vi "mfd_gps.vi"(8 "Refresh Rate (Hz)":u32=5) -> ()   [LabVIEW 2023]
uses:
  mfd_global.vi
panel:
  out "x .or. y?":bool
  out "GPS_RAW_INT":T1
  out "MFD_Gps":picture
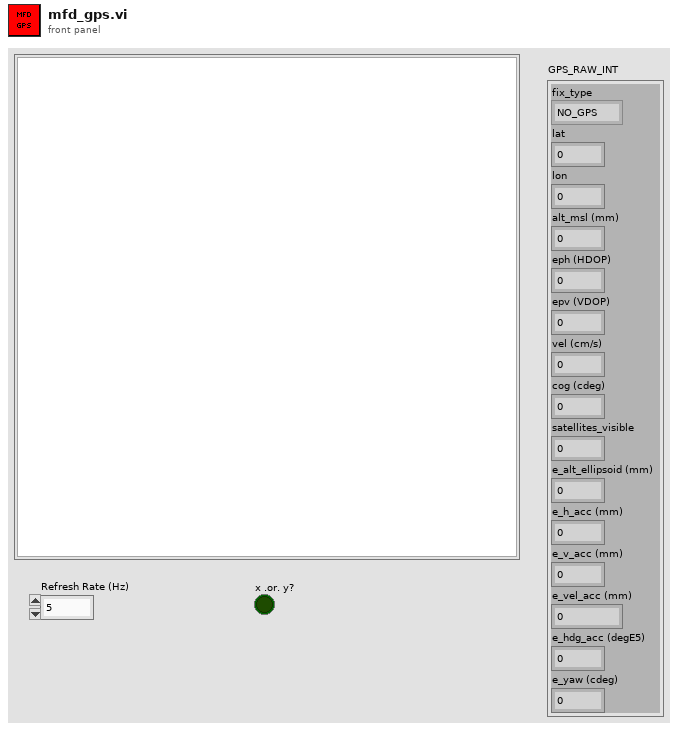
[diagram p1: front panel]
types:
  T1 = cluster{"lat":i32, "lon":i32, "alt_msl (mm)":i32, "eph (HDOP)":u16, "epv (VDOP)":u16, "vel (cm/s)":u16, "cog (cdeg)":u16, "satellites_visible":u8, "e_alt_ellipsoid (mm)":i32, "e_h_acc (mm)":u32, "e_v_acc (mm)":u32, "e_vel_acc (mm)":u32, "e_hdg_acc (degE5)":u32, "e_yaw (cdeg)":u16, "fix_type":enum16{"NO_GPS", "NO_FIX", "2D_FIX", "3D_FIX", "DGPS", "RTK_FLOAT", "RTK_FIXED", "STATIC", "PPP"}}
  T2 = cluster{"left":i16, "top":i16, "right":i16, "bottom":i16}
  T3 = cluster{"Font Name:":string, "Size":i16, "Strikeout?":bool, "Italic?":bool, "Underline?":bool, "Outline?":bool, "Shadow?":bool, "Bold?":bool}
  T4 = enum16{"User-specified Font", "Application Font", "System Font", "Dialog Font"}
  T5 = cluster{"horizontal":enum16{"left", "center", "right"}, "vertical":enum16{"top", "center", "bottom"}}
  T6 = cluster{"Width":u16, "Style":enum32{"Solid", "Dash", "Dot", "DashDot", "DashDotDot"}}
  T7 = typedef "imagedata.ctl" = cluster{"image type":i32, "image depth":i32, "image":u8[], "mask":u8[], "colors":u32[], "Rectangle":cluster{"left":i16, "top":i16, "right":i16, "bottom":i16}}
  T8 = cluster{"lat":bool, "lon":bool, "alt_msl (mm)":bool, "eph (HDOP)":bool, "epv (VDOP)":bool, "vel (cm/s)":bool, "cog (cdeg)":bool, "satellites_visible":bool, "e_alt_ellipsoid (mm)":bool, "e_h_acc (mm)":bool, "e_v_acc (mm)":bool, "e_vel_acc (mm)":bool, "e_hdg_acc (degE5)":bool, "e_yaw (cdeg)":bool, "fix_type":bool}
  T9 = enum16{"NO_GPS", "NO_FIX", "2D_FIX", "3D_FIX", "DGPS", "RTK_FLOAT", "RTK_FIXED", "STATIC", "PPP"}
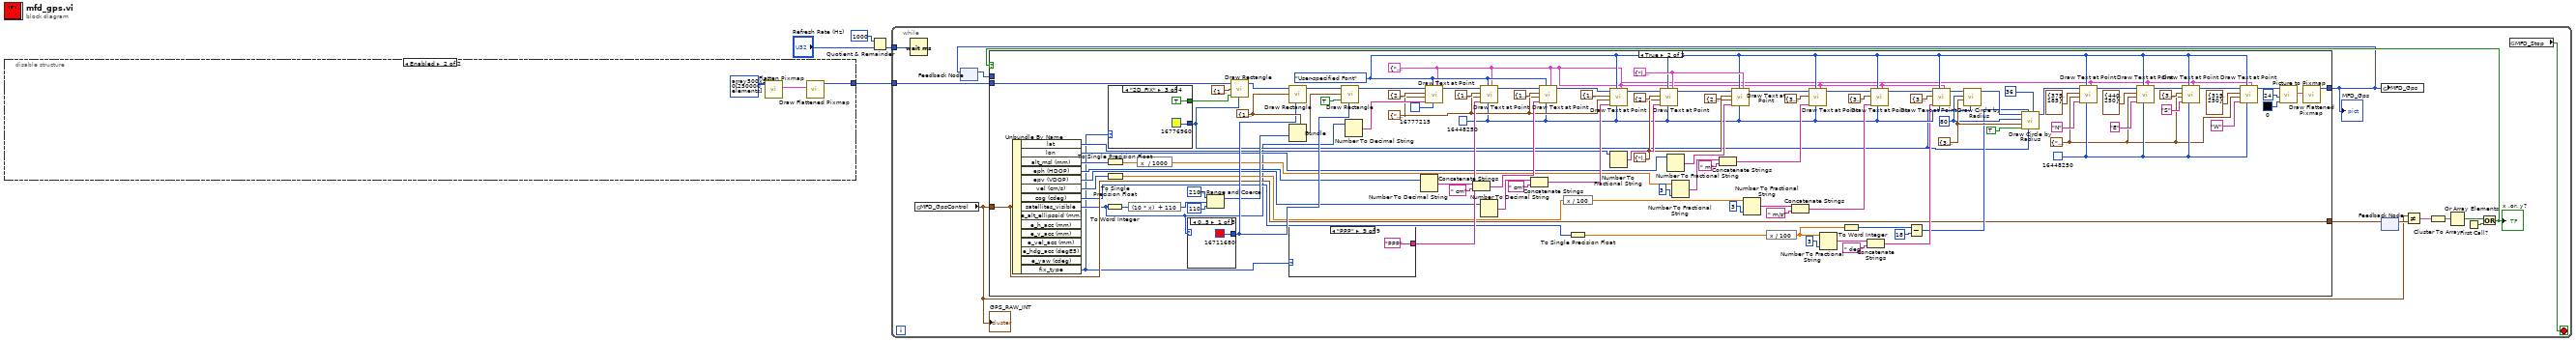
[diagram p0: block diagram]
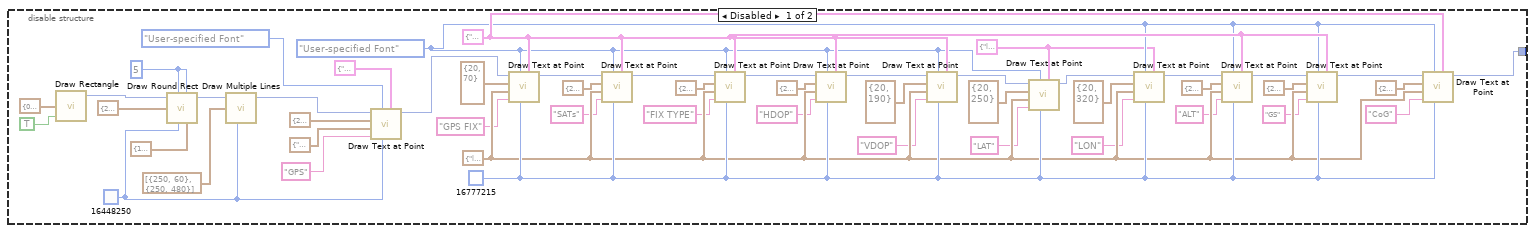
[diagram p2: hidden frame]
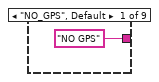
[diagram p4: hidden frame]
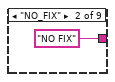
[diagram p5: hidden frame]
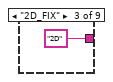
[diagram p6: hidden frame]
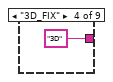
[diagram p7: hidden frame]
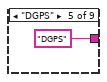
[diagram p8: hidden frame]
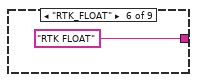
[diagram p9: hidden frame]
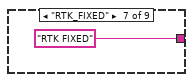
[diagram p10: hidden frame]
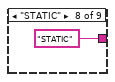
[diagram p11: hidden frame]
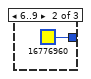
[diagram p12: hidden frame]
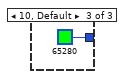
[diagram p13: hidden frame]
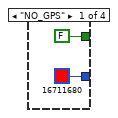
[diagram p14: hidden frame]
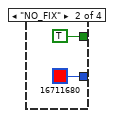
[diagram p15: hidden frame]
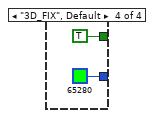
[diagram p16: hidden frame]
diagram:
  n1 = disable-structure shown="Enabled" {
    disable-tunnel: [w5 w56] -> w4
    frame Disabled {
      w32 = T3 {"Font Name:"="latlon", "Size"=21, "Strikeout?"=FALSE, "Italic?"=FALSE, "Underline?"=FALSE, "Outline?"=FALSE, "Shadow?"=FALSE, "Bold?"=TRUE} ("[user-specified font]")
      w38 = T5 {"horizontal"=enum."left", "vertical"=enum."top"} ("alignment(left, top)")
      w42 = T3 {"Font Name:"="gps", "Size"=18, "Strikeout?"=FALSE, "Italic?"=FALSE, "Underline?"=FALSE, "Outline?"=FALSE, "Shadow?"=FALSE, "Bold?"=TRUE} ("[user-specified font]")
      w41 = u32 16777215 ("text color(black)")
      w40 = T4."User-specified Font" ("desired font(Application)")
      w16 = u32 16448250 ("text color(black)")
      w10 = i16 5 ("oval height")
      n2 = call <vilib>:"Draw Rectangle.vi"("rect"=T2 {"left"=0, "top"=0, "right"=500, "bottom"=500}, "fill?(F)"=TRUE) -> ("new picture"=w43:picture)  [unwired: 7 in]
      n3 = call <vilib>:"Draw Round Rect.vi"("picture"=w43, "oval width"=w10, "rect"=T2 {"left"=220, "top"=17, "right"=280, "bottom"=47} ("rect 2"), "color(black)"=w16, "oval height"=w10, "pen"=T6 {"Width"=1, "Style"=enum."Solid"}) -> ("new picture"=w44:picture)  [unwired: 3 in]
      n4 = call <vilib>:"Draw Multiple Lines.vi"("picture"=w44, "line endpoints"=cluster{"x":i16, "y":i16}[] [{"x"=250, "y"=60}, {"x"=250, "y"=480}], "color(black)"=w16) -> ("new picture"=w45:picture)  [unwired: 6 in]
      n5 = call <vilib>:"Draw Text at Point.vi"("[user-specified font]"=T3 {"Font Name:"="r", "Size"=25, "Strikeout?"=FALSE, "Italic?"=FALSE, "Underline?"=FALSE, "Outline?"=FALSE, "Shadow?"=FALSE, "Bold?"=TRUE}, "text color(black)"=w16, "desired font(Application)"=T4."User-specified Font", "text"="GPS", "alignment(left, top)"=T5 {"horizontal"=enum."center", "vertical"=enum."top"}, "origin"=cluster{"x":i16, "y":i16} {"x"=250, "y"=20}, "picture"=w45) -> ("new picture"=w46:picture)  [unwired: 3 in, 1 out]
      n6 = call <vilib>:"Draw Text at Point.vi"("[user-specified font]"=w42, "text color(black)"=w41, "desired font(Application)"=w40, "text"="GPS FIX", "alignment(left, top)"=w38, "origin"=cluster{"x":i16, "y":i16} {"x"=20, "y"=70}, "picture"=w46) -> ("new picture"=w47:picture)  [unwired: 3 in, 1 out]
      n7 = call <vilib>:"Draw Text at Point.vi"("[user-specified font]"=w42, "text color(black)"=w41, "desired font(Application)"=w40, "text"="SATs", "alignment(left, top)"=w38, "origin"=cluster{"x":i16, "y":i16} {"x"=20, "y"=100}, "picture"=w47) -> ("new picture"=w48:picture)  [unwired: 3 in, 1 out]
      n8 = call <vilib>:"Draw Text at Point.vi"("[user-specified font]"=w42, "text color(black)"=w41, "desired font(Application)"=w40, "text"="FIX TYPE", "alignment(left, top)"=w38, "origin"=cluster{"x":i16, "y":i16} {"x"=20, "y"=130} ("origin 2"), "picture"=w48) -> ("new picture"=w49:picture)  [unwired: 3 in, 1 out]
      n9 = call <vilib>:"Draw Text at Point.vi"("[user-specified font]"=w42, "text color(black)"=w41, "desired font(Application)"=w40, "text"="HDOP", "alignment(left, top)"=w38, "origin"=cluster{"x":i16, "y":i16} {"x"=20, "y"=160}, "picture"=w49) -> ("new picture"=w50:picture)  [unwired: 3 in, 1 out]
      n10 = call <vilib>:"Draw Text at Point.vi"("[user-specified font]"=w42, "text color(black)"=w41, "desired font(Application)"=w40, "text"="VDOP", "alignment(left, top)"=w38, "origin"=cluster{"x":i16, "y":i16} {"x"=20, "y"=190}, "picture"=w50) -> ("new picture"=w51:picture)  [unwired: 3 in, 1 out]
      n11 = call <vilib>:"Draw Text at Point.vi"("[user-specified font]"=w32, "text color(black)"=w41, "desired font(Application)"=w40, "text"="LAT", "alignment(left, top)"=w38, "origin"=cluster{"x":i16, "y":i16} {"x"=20, "y"=250}, "picture"=w51) -> ("new picture"=w52:picture)  [unwired: 3 in, 1 out]
      n12 = call <vilib>:"Draw Text at Point.vi"("[user-specified font]"=w32, "text color(black)"=w41, "desired font(Application)"=w40, "text"="LON", "alignment(left, top)"=w38, "origin"=cluster{"x":i16, "y":i16} {"x"=20, "y"=320}, "picture"=w52) -> ("new picture"=w53:picture)  [unwired: 3 in, 1 out]
      n13 = call <vilib>:"Draw Text at Point.vi"("[user-specified font]"=w42, "text color(black)"=w41, "desired font(Application)"=w40, "text"="ALT", "alignment(left, top)"=w38, "origin"=cluster{"x":i16, "y":i16} {"x"=270, "y"=70}, "picture"=w53) -> ("new picture"=w54:picture)  [unwired: 3 in, 1 out]
      n14 = call <vilib>:"Draw Text at Point.vi"("[user-specified font]"=w42, "text color(black)"=w41, "desired font(Application)"=w40, "text"="GS", "alignment(left, top)"=w38, "origin"=cluster{"x":i16, "y":i16} {"x"=270, "y"=100}, "picture"=w54) -> ("new picture"=w55:picture)  [unwired: 3 in, 1 out]
      n15 = call <vilib>:"Draw Text at Point.vi"("[user-specified font]"=w42, "text color(black)"=w41, "desired font(Application)"=w40, "text"="CoG", "alignment(left, top)"=w38, "origin"=cluster{"x":i16, "y":i16} {"x"=270, "y"=130}, "picture"=w55) -> ("new picture"=w5:picture)  [unwired: 3 in, 1 out]
    }
    frame Enabled {
      n16 = call <vilib>:"Flatten Pixmap.vi"("24-bit pixmap"=u32[][] array500x500[250000 elements]) -> ("image data"=w58:T7)  [unwired: 10 in]
      n17 = call <vilib>:"Draw Flattened Pixmap.vi"("image data"=w58) -> ("new picture"=w56:picture)  [unwired: 8 in]
    }
  }
  n18 = Quotient & Remainder(x=u32 1000, y="Refresh Rate (Hz)") -> (floor(x/y)=w1:u32)  [unwired: 1 out]
  n19 = while {
    tunnel: w4 -> [w71]
    tunnel: w1 -> [w70]
    stop <- w61 stop-if-true
    n20 = Wait (ms)(milliseconds to wait=w70) -> ()  [unwired: 1 out]
    n21 = global read "mfd_global.vi" "MFD_GpsControl"() -> (w59:T1)
    "GPS_RAW_INT" <- w59
    n22 = feedback #1() -> (w69:picture)  [unwired: 1 in]
    n23 = feedback #2() -> (w67:T1)  [unwired: 1 in]
    n24 = Not Equal?(x=w59, y=w67) -> (x != y?=w66:T8)
    n25 = Cluster To Array(cluster=w66) -> (array=w65:bool[])
    n26 = Or Array Elements(Boolean array=w65) -> (logical OR=w64:bool)
    n27 = First Call?() -> (First Call?: T/F=w62:bool)
    n28 = Or(x=w64, y=w62) -> (x .or. y?=w63:bool)
    "x .or. y?" <- w63
    n29 = case shown="True" w63 {
      tunnel: w71 -> [_ w179]
      tunnel: w59 -> [w72 w88]
      tunnel: [w73 w74] -> w60
      tunnel: w69 -> [w73 _]
      tunnel: [w72 w88] -> w68
      frame False {
      }
      frame True {
        w89 = T5 {"horizontal"=enum."center", "vertical"=enum."center"} ("alignment(left, top)")
        w90 = u32 16448250 ("text color(black)")
        w111 = cluster{"horizontal":i16, "vertical":i16} {"horizontal"=375, "vertical"=250} ("pixel center")
        w110 = i16 80 ("radius")
        w141 = T3 {"Font Name:"="latlon", "Size"=21, "Strikeout?"=FALSE, "Italic?"=FALSE, "Underline?"=FALSE, "Outline?"=FALSE, "Shadow?"=FALSE, "Bold?"=TRUE} ("[user-specified font]")
        w144 = T5 {"horizontal"=enum."left", "vertical"=enum."top"} ("alignment(left, top)")
        w93 = T3 {"Font Name:"="sat", "Size"=17, "Strikeout?"=FALSE, "Italic?"=FALSE, "Underline?"=FALSE, "Outline?"=FALSE, "Shadow?"=FALSE, "Bold?"=TRUE} ("[user-specified font]")
        w121 = u32 16448250 ("text color(black)")
        w131 = T5 {"horizontal"=enum."center", "vertical"=enum."top"} ("alignment(left, top)")
        w168 = T2 {"left"=110, "top"=100, "right"=210, "bottom"=116} ("rect")
        w94 = T4."User-specified Font" ("desired font(Application)")
        n30 = Unbundle By Name(w88) -> ("lat"=w87:i32, "lon"=w86:i32, "alt_msl (mm)"=w85:i32, "eph (HDOP)"=w84:u16, "epv (VDOP)"=w83:u16, "vel (cm/s)"=w82:u16, "cog (cdeg)"=w81:u16, "satellites_visible"=w80:u8, "fix_type"=w79:T9)  [unwired: 6 out]
        n31 = To Word Integer(number=w80) -> (16bit integer=w163:i16)
        n32 = To Single Precision Float(number=w85) -> (single precision float=w137:sgl)
        n33 = To Single Precision Float(number=w82) -> (single precision float=w127:sgl)
        n34 = case shown="\"2D_FIX\"" w79 {
          tunnel: [FALSE ("fill?(F)") TRUE ("fill?(F)") TRUE ("fill?(F)") TRUE ("fill?(F)")] -> w177
          tunnel: [u32 16711680 ("color(black)") u32 16711680 ("color(black)") u32 16776960 ("color(black)") u32 65280 ("color(black)")] -> w102
          frame "NO_GPS" {
          }
          frame "NO_FIX" {
          }
          frame "2D_FIX" {
          }
          frame "3D_FIX", Default {
          }
        }
        n35 = expression code="(10 * x)  + 110"(w163) -> (w162:i16)
        n36 = expression code="x  / 1000"(w137) -> (w138:sgl)
        n37 = case shown="0..5" w80 {
          tunnel: [u32 16711680 ("color(black)") u32 16776960 ("color(black)") u32 65280 ("color(black)")] -> w167
          frame 0..5 {
          }
          frame 6..9 {
          }
          frame 10, Default {
          }
        }
        n38 = In Range and Coerce(upper limit=i16 210, x=w162, lower limit=i16 110) -> (coerced(x)=w166:i16)  [unwired: 1 out]
        n39 = call <vilib>:"Draw Rectangle.vi"("picture"=w179, "rect"=T2 {"left"=110, "top"=70, "right"=210, "bottom"=86}, "fill?(F)"=w177, "color(black)"=w102) -> ("new picture"=w170:picture)  [unwired: 5 in]
        n40 = call <vilib>:"Draw Rectangle.vi"("picture"=w170, "rect"=w168, "color(black)"=w167) -> ("new picture"=w169:picture)  [unwired: 6 in]
        n41 = Bundle(cluster=w168, "right"=w166) -> (w171:T2)  [unwired: 3 in]
        n42 = case shown="\"PPP\"" w79 {
          tunnel: ["NO GPS" "NO FIX" "2D" "3D" "DGPS" "RTK FLOAT" "RTK FIXED" "STATIC" "PPP"] -> w159
          frame "NO_GPS", Default {
          }
          frame "NO_FIX" {
          }
          frame "2D_FIX" {
          }
          frame "3D_FIX" {
          }
          frame "DGPS" {
          }
          frame "RTK_FLOAT" {
          }
          frame "RTK_FIXED" {
          }
          frame "STATIC" {
          }
          frame "PPP" {
          }
        }
        n43 = call <vilib>:"Draw Rectangle.vi"("picture"=w169, "rect"=w171, "fill?(F)"=TRUE, "color(black)"=w167) -> ("new picture"=w175:picture)  [unwired: 5 in]
        n44 = Number To Decimal String(number=w80) -> (decimal integer string=w173:string)  [unwired: 1 in]
        n45 = Number To Decimal String(number=w84) -> (decimal integer string=w156:string)  [unwired: 1 in]
        n46 = call <vilib>:"Draw Text at Point.vi"("[user-specified font]"=w93, "text color(black)"=u32 16777215, "desired font(Application)"=w94, "text"=w173, "alignment(left, top)"=w131, "origin"=cluster{"x":i16, "y":i16} {"x"=231, "y"=100}, "picture"=w175) -> ("new picture"=w161:picture)  [unwired: 3 in, 1 out]
        n47 = Concatenate Strings(w156, " cm" ("string")) -> (w155:string)
        n48 = call <vilib>:"Draw Text at Point.vi"("[user-specified font]"=w93, "text color(black)"=w121, "desired font(Application)"=w94, "text"=w159, "alignment(left, top)"=w131, "origin"=cluster{"x":i16, "y":i16} {"x"=160, "y"=130}, "picture"=w161) -> ("new picture"=w158:picture)  [unwired: 3 in, 1 out]
        n49 = Number To Decimal String(number=w83) -> (decimal integer string=w151:string)  [unwired: 1 in]
        n50 = Concatenate Strings(w151, " cm" ("string")) -> (w149:string)
        n51 = call <vilib>:"Draw Text at Point.vi"("[user-specified font]"=w93, "text color(black)"=w121, "desired font(Application)"=w94, "text"=w155, "alignment(left, top)"=w131, "origin"=cluster{"x":i16, "y":i16} {"x"=160, "y"=160}, "picture"=w158) -> ("new picture"=w153:picture)  [unwired: 3 in, 1 out]
        n52 = expression code="x / 100"(w127) -> (w126:sgl)
        n53 = To Single Precision Float(number=w81) -> (single precision float=w120:sgl)
        n54 = call <vilib>:"Draw Text at Point.vi"("[user-specified font]"=w93, "text color(black)"=w121, "desired font(Application)"=w94, "text"=w149, "alignment(left, top)"=w131, "origin"=cluster{"x":i16, "y":i16} {"x"=160, "y"=190} ("origin 2"), "picture"=w153) -> ("new picture"=w148:picture)  [unwired: 3 in, 1 out]
        n55 = Number To Fractional String(number=w87) -> (F-format string=w146:string)  [unwired: 3 in]
        n56 = call <vilib>:"Draw Text at Point.vi"("[user-specified font]"=w141, "text color(black)"=w121, "desired font(Application)"=w94, "text"=w146, "alignment(left, top)"=w144, "origin"=cluster{"x":i16, "y":i16} {"x"=20, "y"=280} ("origin 2"), "picture"=w148) -> ("new picture"=w145:picture)  [unwired: 3 in, 1 out]
        n57 = Number To Fractional String(number=w86) -> (F-format string=w142:string)  [unwired: 3 in]
        n58 = Number To Fractional String(number=w138, precision (6)=i16 3) -> (F-format string=w135:string)  [unwired: 2 in]
        n59 = Concatenate Strings(w135, " m" ("string")) -> (w134:string)
        n60 = call <vilib>:"Draw Text at Point.vi"("[user-specified font]"=w141, "text color(black)"=w121, "desired font(Application)"=w94, "text"=w142, "alignment(left, top)"=w144, "origin"=cluster{"x":i16, "y":i16} {"x"=20, "y"=350} ("origin 3"), "picture"=w145) -> ("new picture"=w140:picture)  [unwired: 3 in, 1 out]
        n61 = Number To Fractional String(number=w126, precision (6)=i16 3) -> (F-format string=w125:string)  [unwired: 2 in]
        n62 = expression code="x / 100"(w120) -> (w109:sgl)
        n63 = Concatenate Strings(w125, " m/s" ("string")) -> (w128:string)
        n64 = call <vilib>:"Draw Text at Point.vi"("[user-specified font]"=w93, "text color(black)"=w121, "desired font(Application)"=w94, "text"=w134, "origin"=cluster{"x":i16, "y":i16} {"x"=340, "y"=70} ("origin 2"), "picture"=w140) -> ("new picture"=w132:picture)  [unwired: 4 in, 1 out]
        n65 = Number To Fractional String(number=w109, precision (6)=i16 3) -> (F-format string=w117:string)  [unwired: 2 in]
        n66 = To Word Integer(number=w109) -> (16bit integer=w107:i16)
        n67 = Concatenate Strings(w117, " deg" ("string")) -> (w116:string)
        n68 = call <vilib>:"Draw Text at Point.vi"("[user-specified font]"=w93, "text color(black)"=w121, "desired font(Application)"=w94, "text"=w128, "origin"=cluster{"x":i16, "y":i16} {"x"=340, "y"=100}, "picture"=w132) -> ("new picture"=w123:picture)  [unwired: 4 in, 1 out]
        n69 = Subtract(x=w107, y=i16 18) -> (x-y=w106:i16)
        n70 = call <vilib>:"Draw Text at Point.vi"("[user-specified font]"=w93, "text color(black)"=w121, "desired font(Application)"=w94, "text"=w116, "origin"=cluster{"x":i16, "y":i16} {"x"=340, "y"=130}, "picture"=w123) -> ("new picture"=w115:picture)  [unwired: 4 in, 1 out]
        n71 = call <vilib>:"Draw Circle by Radius.vi"("color(black)"=w102, "pixel center"=w111, "radius"=w110, "picture"=w115) -> ("new picture"=w114:picture)  [unwired: 7 in]
        n72 = call <vilib>:"Draw Circle by Radius.vi"("arc size(360)"=i16 36, "color(black)"=w102, "start angle(0)"=w106, "fill?(F)"=TRUE, "pixel center"=w111, "radius"=w110, "picture"=w114) -> ("new picture"=w105:picture)  [unwired: 4 in]
        n73 = call <vilib>:"Draw Text at Point.vi"("[user-specified font]"=w93, "text color(black)"=w90, "desired font(Application)"=w94, "text"="N", "alignment(left, top)"=w89, "origin"=cluster{"x":i16, "y":i16} {"x"=375, "y"=185}, "picture"=w105) -> ("new picture"=w101:picture)  [unwired: 3 in, 1 out]
        n74 = call <vilib>:"Draw Text at Point.vi"("[user-specified font]"=w93, "text color(black)"=w90, "desired font(Application)"=w94, "text"="E", "alignment(left, top)"=w89, "origin"=cluster{"x":i16, "y":i16} {"x"=440, "y"=250} ("origin 2"), "picture"=w101) -> ("new picture"=w98:picture)  [unwired: 3 in, 1 out]
        n75 = call <vilib>:"Draw Text at Point.vi"("[user-specified font]"=w93, "text color(black)"=w90, "desired font(Application)"=w94, "text"="S", "alignment(left, top)"=w89, "origin"=cluster{"x":i16, "y":i16} {"x"=375, "y"=315}, "picture"=w98) -> ("new picture"=w95:picture)  [unwired: 3 in, 1 out]
        n76 = call <vilib>:"Draw Text at Point.vi"("[user-specified font]"=w93, "text color(black)"=w90, "desired font(Application)"=w94, "text"="W", "alignment(left, top)"=w89, "origin"=cluster{"x":i16, "y":i16} {"x"=315, "y"=250}, "picture"=w95) -> ("new picture"=w75:picture)  [unwired: 3 in, 1 out]
        n77 = call <vilib>:"Picture to Pixmap.vi"("Background Color"=u32 0, "depth"=24, "picture"=w75) -> ("image data"=w78:T7)  [unwired: 7 in, 1 out]
        n78 = call <vilib>:"Draw Flattened Pixmap.vi"("image data"=w78) -> ("new picture"=w74:picture)  [unwired: 8 in]
      }
    }
    "MFD_Gps" <- w60
    n79 = feedback-in #1(w60) -> ()
    n80 = global write "mfd_global.vi" "MFD_Gps"(w60) -> ()
    n81 = feedback-in #2(w68) -> ()
    n82 = global read "mfd_global.vi" "MFD_Stop"() -> (w61:bool)
  }
